vi "init request string.vi"(8 "error in (no error)":errorcluster, 10 "slsc type":T1, 11 "resource":string) -> (0 "error out":errorcluster, 3 "Request String":string)   [LabVIEW 2015, in "SLSC Remote.lvclass"]
uses:
  SLSC Remote.lvclass
  SLSC Interface Class/slsc type.ctl
  <vilib>/NI/i3 JSON/JSON Generation/Create Value Files/Create Value - Object.vi
  <vilib>/NI/i3 JSON/JSON Generation/Add Object Parameter Files/Add Object Parameter - String.vi
  <vilib>/NI/NI JSONRPC Server Framework/Classes/Server/Format Client Request (Auto-Increment).vi
  <vilib>/NI/i3 JSON/i3-json.lvlib
  <vilib>/NI/NI JSONRPC Server Framework/Classes/Server/JSONRPC Server.lvclass
  SLSC Interface Class/SLSC Interface.lvclass
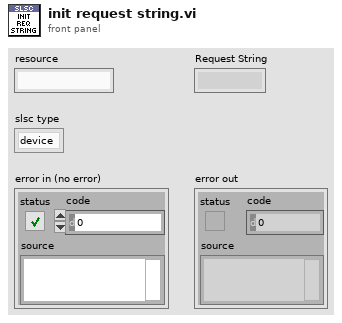
[diagram p1: front panel]
types:
  T1 = typedef "SLSC Interface.lvclass/slsc type.ctl" = enum16{"device", "nvmem", "channel", "none"}
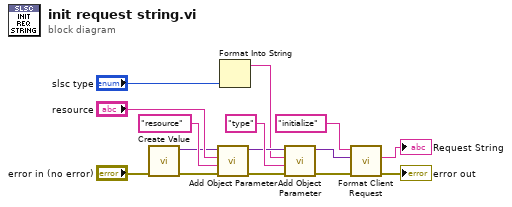
[diagram p0: block diagram]
diagram:
  n1 = call-poly <vilib>:"Create Value.vi"("error in (no error)"="error in (no error)") -> ("error out"=w6:errorcluster, "JSON Tree"=w3:variant)  [unwired: 9 in]
  n2 = call-poly <vilib>:"Add Object Parameter.vi"("error in (no error)"=w6, "Name"="resource", "String"="resource", "JSON Tree in (JSON Object)"=w3) -> ("error out"=w5:errorcluster, "JSON Tree out (JSON Object)"=w4:variant)  [unwired: 6 in]
  n3 = Format Into String("slsc type") -> (resulting string=w1:string)  [unwired: 3 in, 1 out]
  n4 = call-poly <vilib>:"Add Object Parameter.vi"("error in (no error)"=w5, "Name"="type", "String"=w1, "JSON Tree in (JSON Object)"=w4) -> ("error out"=w12:errorcluster, "JSON Tree out (JSON Object)"=w10:variant)  [unwired: 6 in]
  n5 = call-poly <vilib>:"Format Client Request.vi"("error in (no error)"=w12, "params"=w10, "method"="initialize") -> ("error out"=→"error out":errorcluster, "Request String"=→"Request String":string)  [unwired: 7 in]
